vi "init.vi"(8 "error in (no error)":errorcluster, 11 "B in":refnum<class "B.lvclass">) -> (0 "error out":errorcluster, 3 "B out":refnum<class "B.lvclass">)   [LabVIEW 2015, in "B.lvclass"]
uses:
  B.lvclass
  General.lvclass
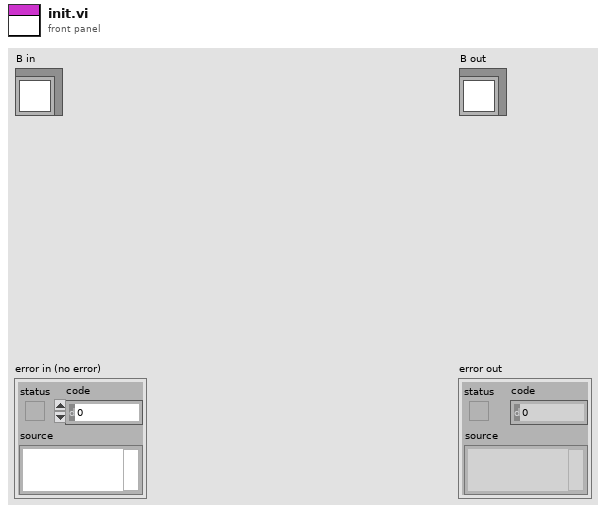
[diagram p1: front panel]
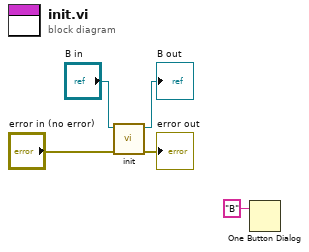
[diagram p0: block diagram]
diagram:
  n1 = call-parent "init.vi"("error in (no error)"="error in (no error)", "General in"="B in") -> ("error out"=→"error out":errorcluster, "General out"=→"B out":refnum<class "B.lvclass">)  [unwired: 8 in]
  n2 = One Button Dialog(message="B") -> ()  [unwired: 1 in, 1 out]
